vi "Tag_Buffer_Dbl_VIG.vi"(7 "Operation":enum16{"get data", "set data", "initialize"}(ring)=enum."set data", 8 "error in":errorcluster, 10 "tag_names_in":string[](array[string]), 11 "tag_data_in":dbl[](array[numeric])) -> (0 "error out":errorcluster, 2 "tag_names_out":string[](array[string]), 3 "tag_data_out":dbl[](array[numeric]))   [LabVIEW 2010]
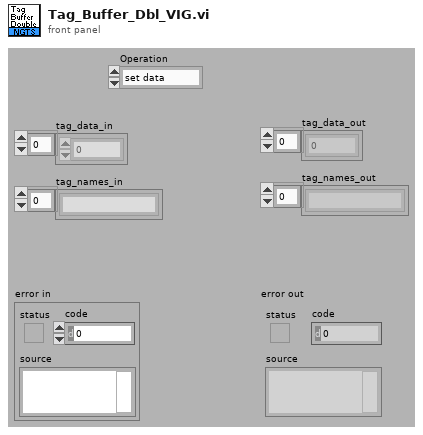
[diagram p1: front panel]
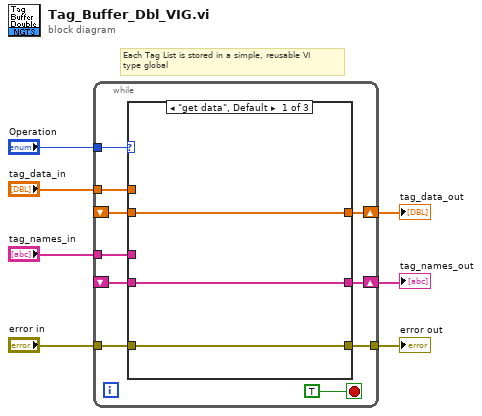
[diagram p0: block diagram]
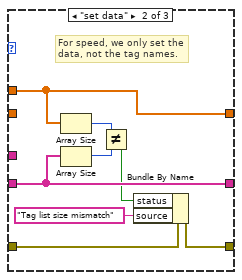
[diagram p2: hidden frame]
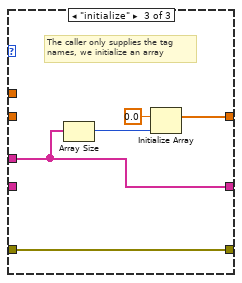
[diagram p3: hidden frame]
diagram:
  # "Each Tag List is stored in a simple, reusable VI\ntype global"
  n1 = while {
    tunnel: "Operation" -> [w17]
    shift-right: [w15] -> w5
    shift-left: _ -> [w13]
    tunnel: "tag_data_in" -> [w14]
    shift-right: [w11] -> w3
    shift-left: _ -> [w10]
    tunnel: "tag_names_in" -> [w12]
    tunnel: "error in" -> [w9]
    tunnel: [w8] -> w1
    stop <- TRUE stop-if-true
    n2 = case shown="\"get data\", Default" w17 {
      tunnel: [w20 w28 w31] -> w15
      tunnel: w14 -> [_ w28 _]
      tunnel: w13 -> [w20 _ _]
      tunnel: w12 -> [_ _ w33]
      tunnel: [w19 w27 w33] -> w11
      tunnel: w10 -> [w19 w27 _]
      tunnel: w9 -> [w18 w24 w30]
      tunnel: [w18 w23 w30] -> w8
      frame "get data", Default {
      }
      frame "set data" {
        # "For speed, we only set the\ndata, not the tag names."
        n3 = Array Size(array=w28) -> (size(s)=w25:i32)
        n4 = Array Size(array=w27) -> (size(s)=w26:i32)
        n5 = Not Equal?(x=w25, y=w26) -> (x != y?=w22:bool)
        n6 = Bundle By Name(cluster=w24, "status"=w22, "source"="Tag list size mismatch") -> (w23:errorcluster)
      }
      frame "initialize" {
        # "The caller only supplies the tag\nnames, we initialize an array"
        n7 = Array Size(array=w33) -> (size(s)=w32:i32)
        n8 = Initialize Array(0.0 ("element"), w32) -> (w31:dbl[])
      }
    }
  }
  "error out" <- w1
  "tag_data_out" <- w5
  "tag_names_out" <- w3
